vi "YKMW100 Write Com Register.vi"(0 "VISA session":refnum<visa-resource-name>="MW100", 5 "Channel":string="C001", 7 "Value":string="000", 11 "error in (no error)":errorcluster, 12 "Debug":bool) -> (4 "dup VISA session":refnum<visa-resource-name>="MW100", 15 "error out":errorcluster)   [LabVIEW 2020]
panel:
  out "CMD":string
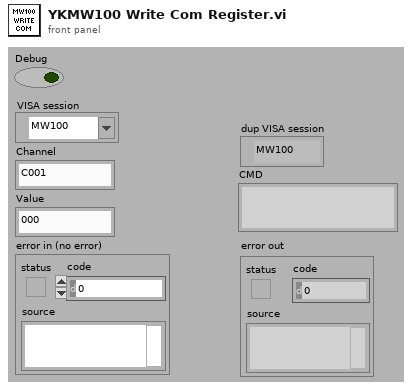
[diagram p1: front panel]
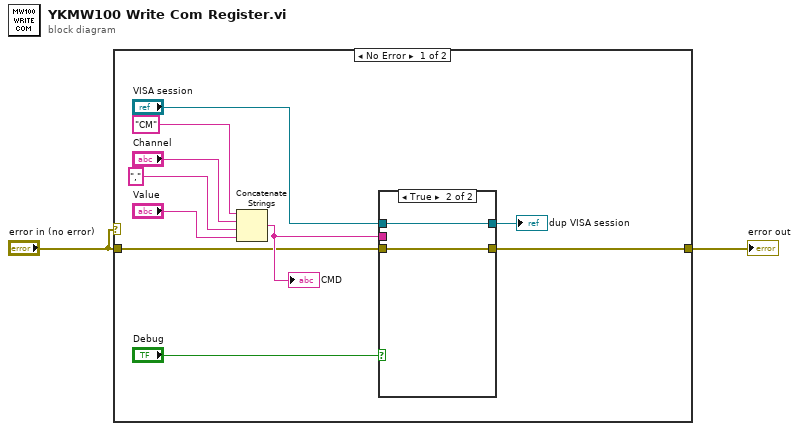
[diagram p0: block diagram]
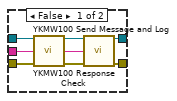
[diagram p2: hidden frame]
diagram:
  n1 = case shown="No Error" "error in (no error)" {
    selector: "error in (no error)" -> [_ w23]
    tunnel: [w4 w23] -> w2
    tunnel: "error in (no error)" -> [w5 _]
    frame No Error {
      n2 = Concatenate Strings("CM" ("string"), "Channel", "," ("string"), "Value") -> (w6:string)
      "CMD" <- w6
      n3 = case shown="True" "Debug" {
        tunnel: [w17 w22] -> w12
        tunnel: "VISA session" -> [w16 w22]
        tunnel: w6 -> [w15 _]
        tunnel: w5 -> [w14 w21]
        tunnel: [w13 w21] -> w4
        frame False {
          n4 = call "YKMW100 Send Message and Log.vi"("VISA session"=w16, "Send Message (\"\")"=w15, "error in (no error)"=w14) -> ("dup VISA session"=w20:refnum<visa-resource-name>, "Read Buffer"=w18:string, "error out"=w19:errorcluster)  [unwired: 10 in]
          n5 = call "YKMW100 Response Check.vi"("VISA session"=w20, "Message In (\"\")"=w18, "error in (no error)"=w19) -> ("dup VISA session"=w17:refnum<visa-resource-name>, "error out"=w13:errorcluster)  [unwired: 8 in, 3 out]
        }
        frame True {
        }
      }
      "dup VISA session" <- w12
    }
    frame Error {
    }
  }
  "error out" <- w2
